vi "Connect.vi"(8 "error in (no error)":errorcluster, 9 "timeout (ms)":i32=200, 11 "TCP_Streamer_Subscriber in":refnum<class "TCP_Streamer_Subscriber.lvclass">) -> (0 "error out":errorcluster, 3 "TCP_Streamer_Subscriber out":refnum<class "TCP_Streamer_Subscriber.lvclass">)   [LabVIEW 2021, in "TCP_Streamer_Subscriber.lvclass"]
uses:
  TCP_Streamer_Subscriber.lvclass
  Typedef/State.ctl
  TCP_Streamer_Subscriber.lvclass/TCP_Streamer_Subscriber.ctl
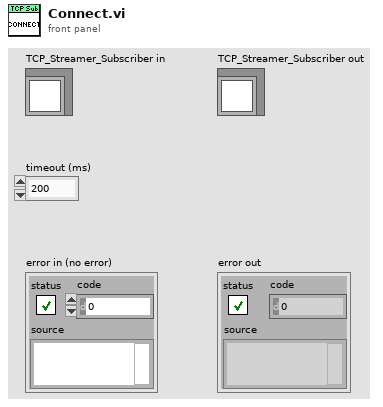
[diagram p1: front panel]
types:
  T1 = typedef "TCP_Streamer_Subscriber.lvclass/State.ctl" = enum16{"Stopped", "Connecting", "Receiving"}
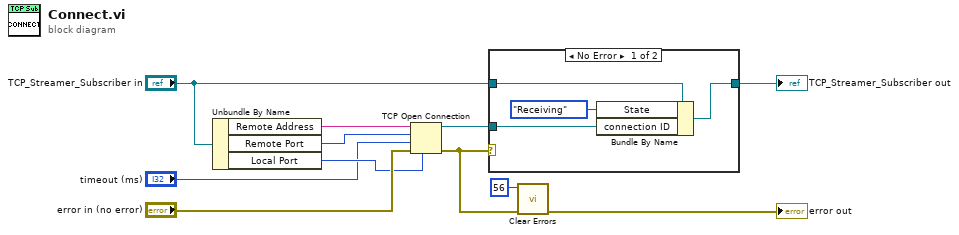
[diagram p0: block diagram]
diagram:
  n1 = Unbundle By Name("TCP_Streamer_Subscriber in") -> ("Remote Address"=w8:string, "Remote Port"=w7:u16, "Local Port"=w6:u16)
  n2 = TCP Open Connection(address=w8, remote port or service name=w7, timeout ms (60000)="timeout (ms)", local port=w6, error in (no error)="error in (no error)") -> (connection ID=w9:refnum<k5>, error out=w4:errorcluster)
  n3 = case shown="No Error" w4 {
    tunnel: "TCP_Streamer_Subscriber in" -> [w15 w16]
    tunnel: [w14 w16] -> w10
    tunnel: w9 -> [w13 _]
    frame No Error {
      n4 = Bundle By Name(cluster=w15, "State"=State."Receiving", "connection ID"=w13) -> (w14:refnum<class "TCP_Streamer_Subscriber.lvclass">)
    }
    frame Error {
    }
  }
  "TCP_Streamer_Subscriber out" <- w10
  n5 = call <vilib>:"Clear Errors.vi"("error in (no error)"=w4, "specific error code to clear (0: all)"=56) -> ("error out"=→"error out":errorcluster)  [unwired: 4 in, 1 out]
